vi "test12-LocalExternalStateRegistration.vi"(8 "error in (no error)":errorcluster, 11 "TestCase in":refnum<class "testcase-CSMBroadcast.lvclass">) -> (0 "error out":errorcluster, 3 "TestCase out":refnum<class "testcase-CSMBroadcast.lvclass">)   [LabVIEW 2017, in "testcase-CSMBroadcast.lvclass"]
uses:
  testcase-CSMBroadcast.lvclass
  0b17d103-e67b-41be-a9eb-a2ee1311ff1f.vi
  5999693e-4f8a-4b34-ae87-f34dff5771be.vi
  52a2a10a-a04b-4bad-8df4-e1eb944f47cc.vi
  826f03dd-b4b5-4c6b-9085-8edf6da4f43b.vi
  src/user.lib/_NEVSTOP/Communicable State Machine(CSM)/AdvanceAPI/CSM - Revert Arguments-Safe String.vi
  src/user.lib/_NEVSTOP/Communicable State Machine(CSM)/AdvanceAPI/CSM - Make String Arguments Safe.vi
  src/user.lib/_NEVSTOP/Communicable State Machine(CSM)/AdvanceAPI/CSM - Break Down Multiple States String.vi
  src/user.lib/_NEVSTOP/Communicable State Machine(CSM)/AdvanceAPI/CSM - Keywords.vi
  src/user.lib/_NEVSTOP/Communicable State Machine(CSM)/_Polymophic/CSM - Replace Marks in Messages.vi
  src/user.lib/_NEVSTOP/Communicable State Machine(CSM)/AdvanceAPI/CSM - Get Module Attribute.vi
  src/user.lib/_NEVSTOP/Communicable State Machine(CSM)/_Shared/Trim Single-line Text.vi
  <vilib>/addons/_JKI Toolkits/VI Tester/TestCase.llb/TestCase.lvclass
  src/user.lib/_NEVSTOP/Communicable State Machine(CSM)/Communicable State Machine.lvlib
  CSM/CSM-Testcase.lvlib
  C:/Program Files (x86)/National Instruments/LabVIEW 2017/vi.lib/addons/_JKI Toolkits/VI Tester/TestCase.llb/TestCase.lvclass
panel:
  out "One-Shot Unregistrations":string
  out "One-Shot Registrations":string
  out "LoopCount 2":i32
  out "State History":string
  out "LoopCount":i32
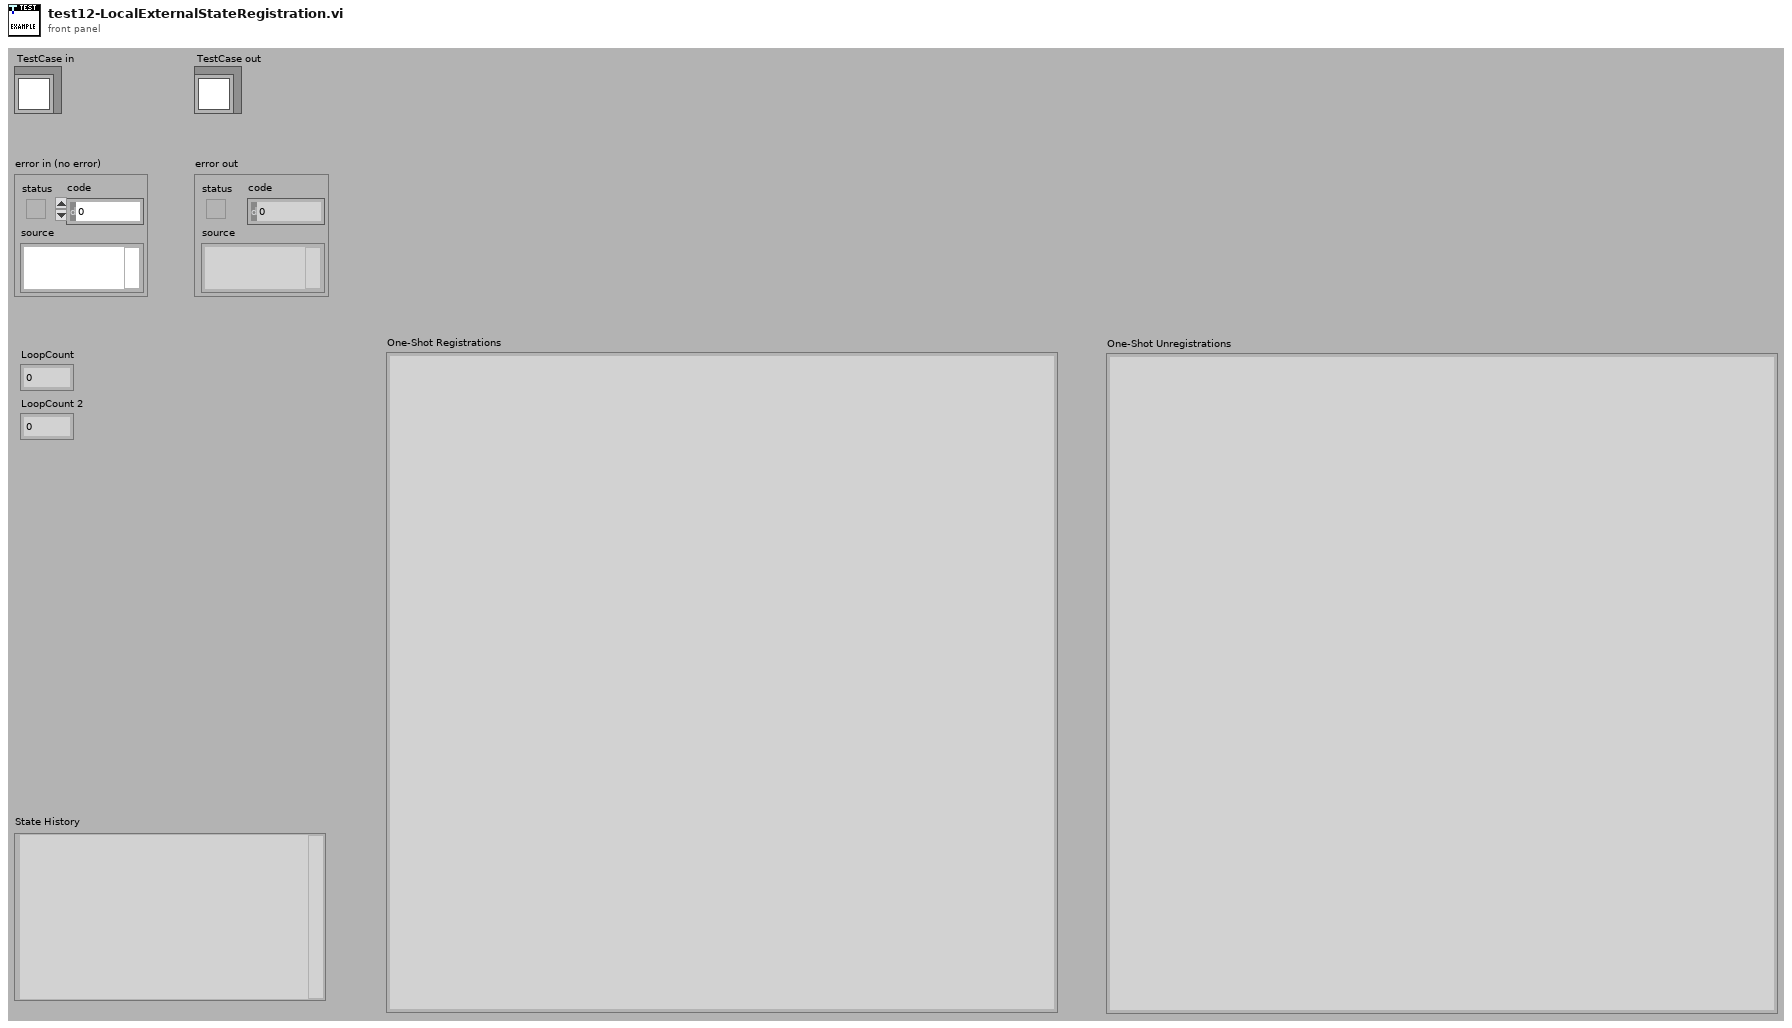
[diagram p1: front panel]
types:
  T1 = enum32{"Invalid", "Standard", "Closed", "Hidden", "Minimized", "Maximized"}
  T2 = enum32{"invalid app kind", "Development System", "Run Time System", "Student Edition", "Embedded LabVIEW", "Evaluation", "Custom"}
  T3 = typedef "Communicable State Machine.lvlib/_CSM_Response Source Message.ctl" = cluster{"‘State":string, "’Arguments":string, "’Error":errorcluster}
  T4 = cluster{"Current VI Reference":refnum<vi>, "Close Panel on Exit?":bool}
  T5 = cluster{"Core":cluster{"Current VI Reference":refnum<vi>, "Close Panel on Exit?":bool}, "Your Boolean data":bool, "Your string data":string}
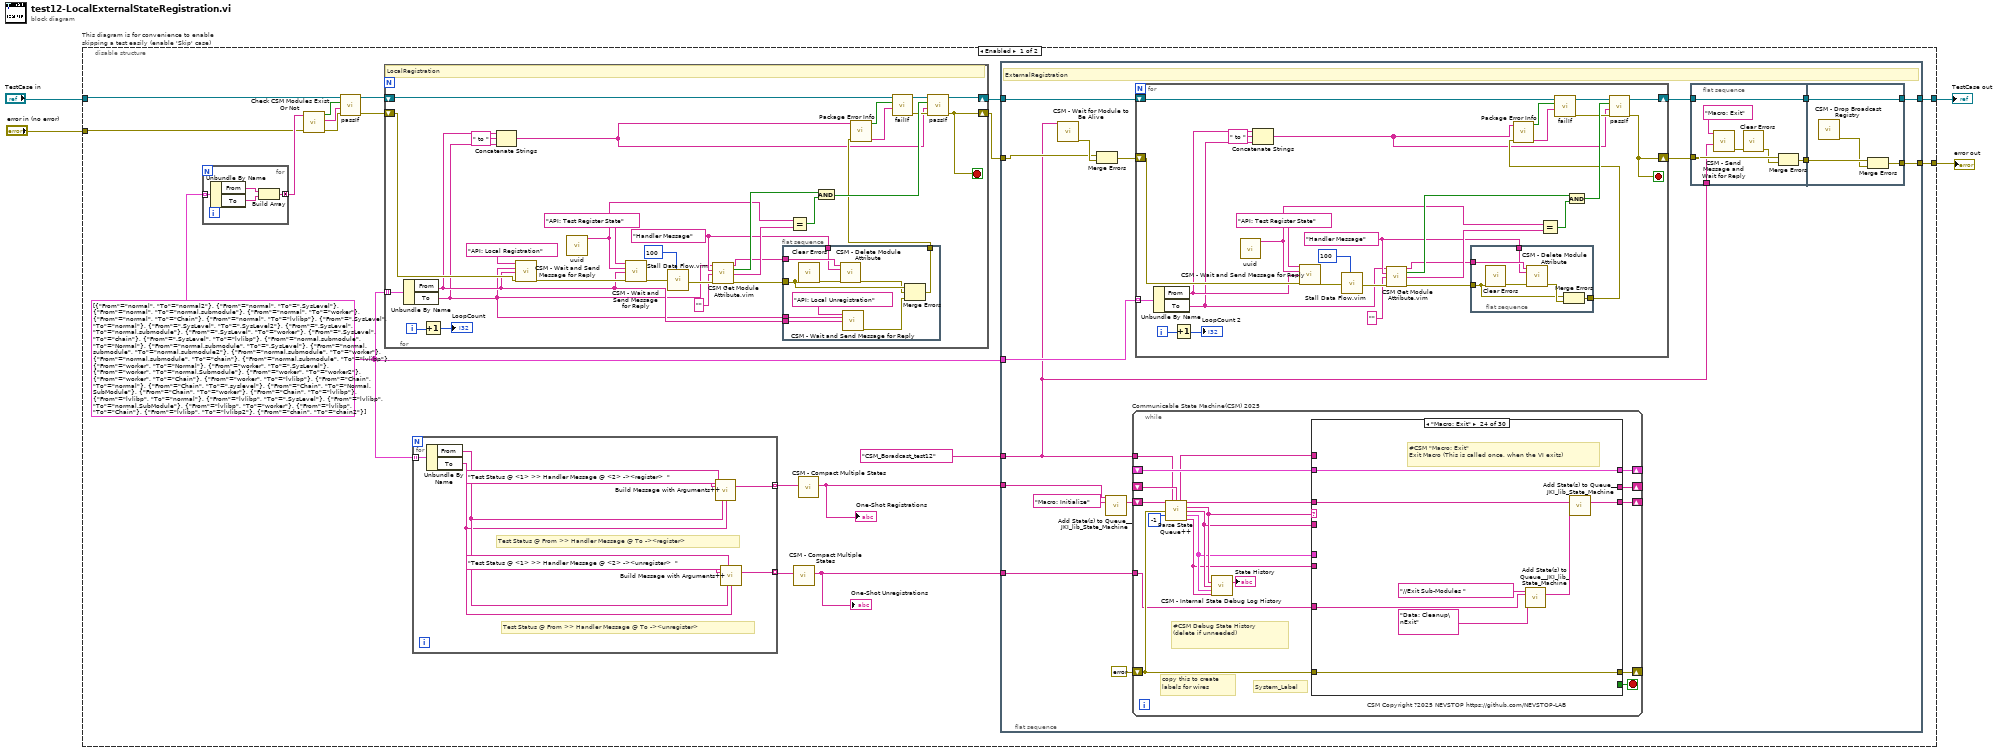
[diagram p0: block diagram]
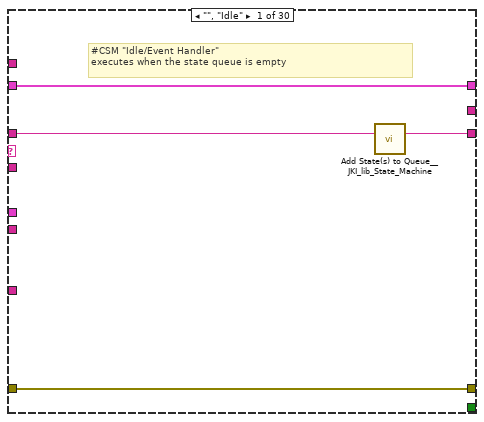
[diagram p2: hidden frame]
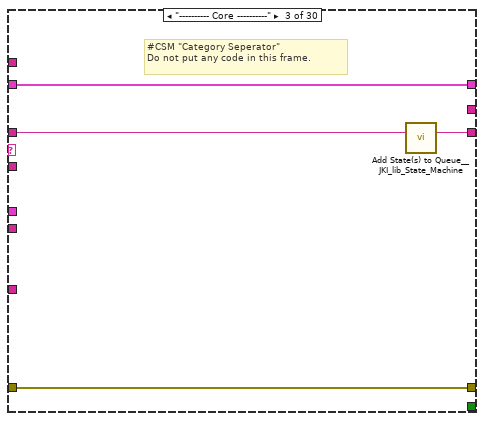
[diagram p4: hidden frame]
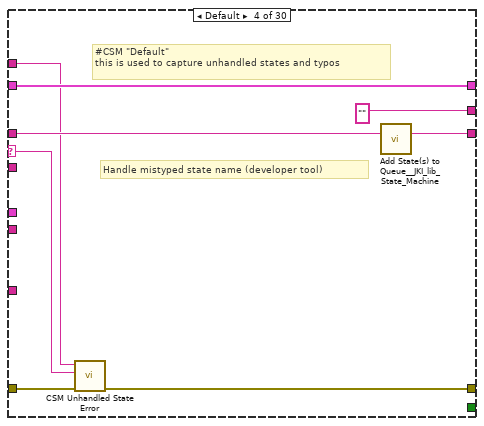
[diagram p5: hidden frame]
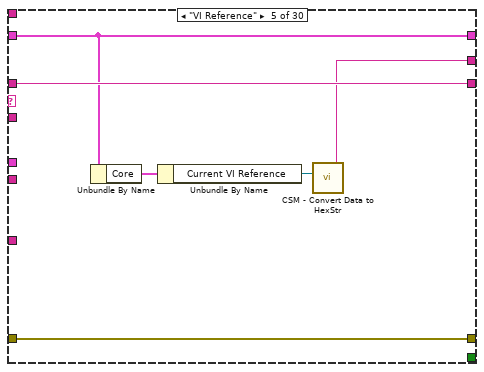
[diagram p6: hidden frame]
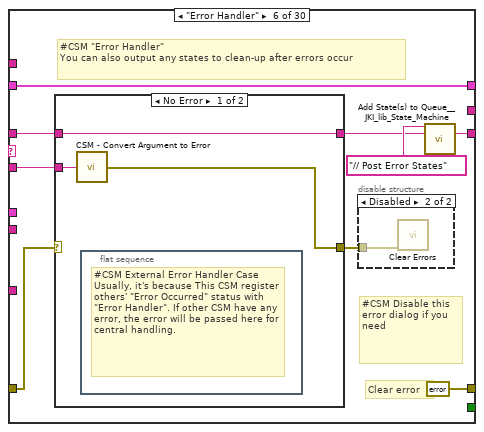
[diagram p7: hidden frame]
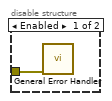
[diagram p8: hidden frame]
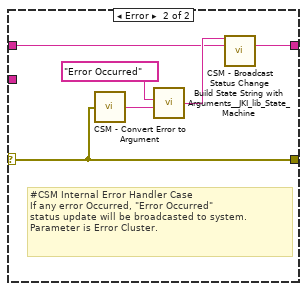
[diagram p9: hidden frame]
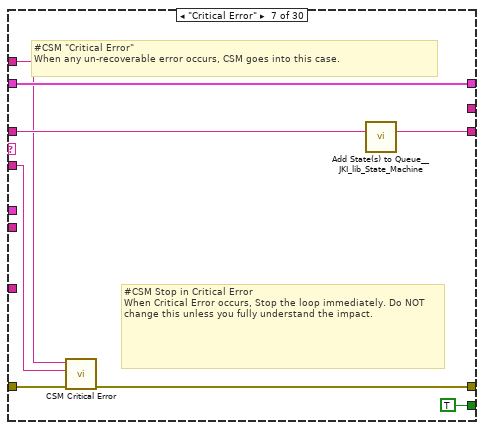
[diagram p10: hidden frame]
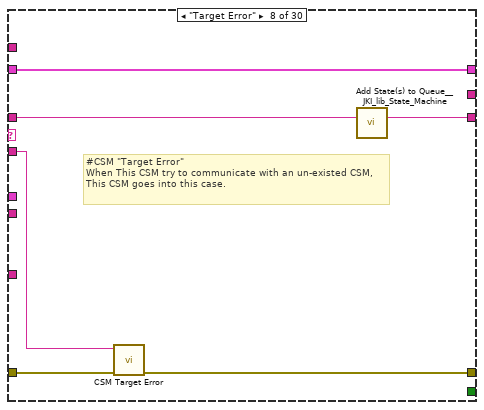
[diagram p11: hidden frame]
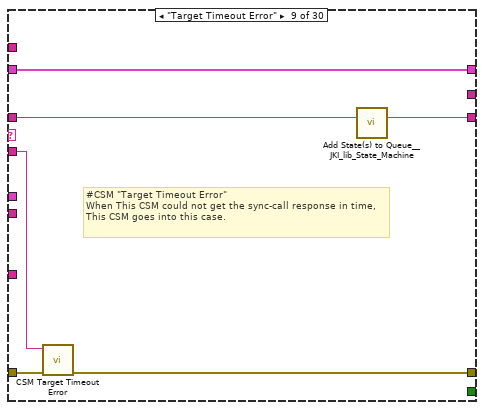
[diagram p12: hidden frame]
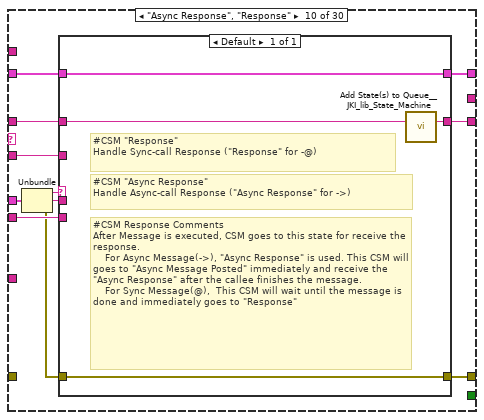
[diagram p13: hidden frame]
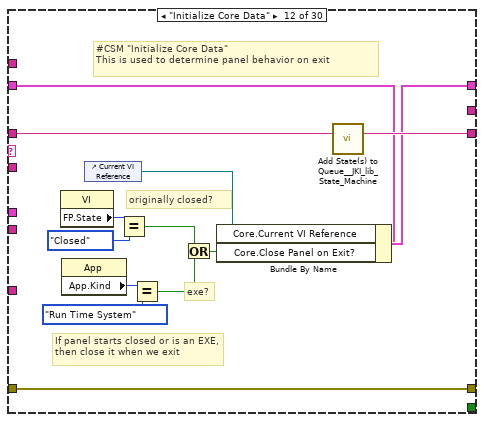
[diagram p15: hidden frame]
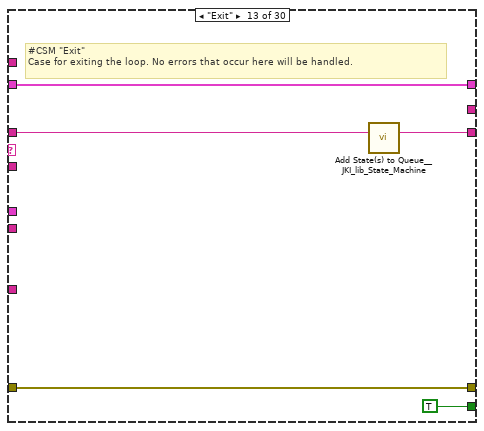
[diagram p16: hidden frame]
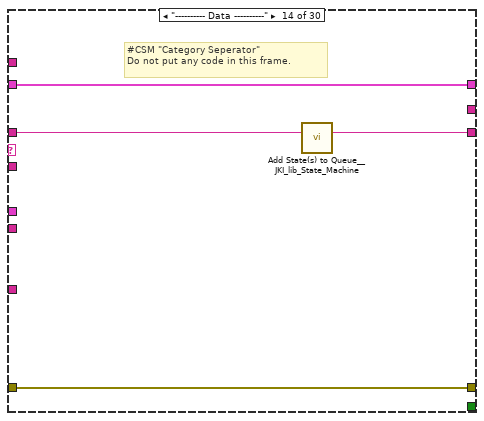
[diagram p17: hidden frame]
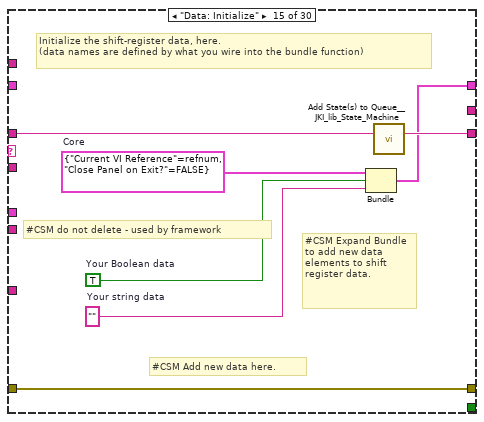
[diagram p18: hidden frame]
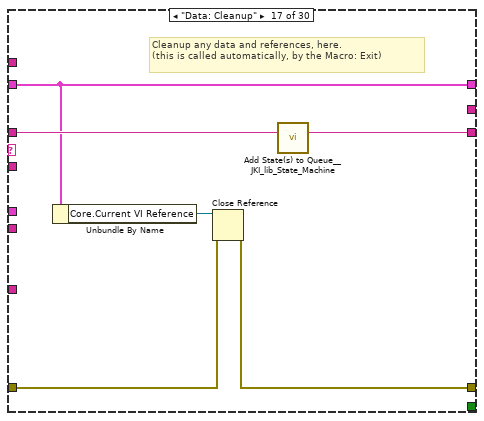
[diagram p20: hidden frame]
diagram:
  n1 = disable-structure "This diagram is for convenience to enable skipping a test easily (enable 'Skip' case)" shown="Enabled" {
    disable-tunnel: "TestCase in" -> [w10 w418]
    disable-tunnel: [w6 w416] -> w1
    disable-tunnel: [w16 w417] -> w3
    disable-tunnel: "error in (no error)" -> [w7 w415]
    frame Enabled {
      w11 = cluster{"From":string, "To":string}[] [{"From"="normal", "To"="normal2"}, {"From"="normal", "To"=".SysLevel"}, {"From"="normal", "To"="normal.submodule"}, {"From"="normal", "To"="worker"}, {"From"="normal", "To"="Chain"}, {"From"="normal", "To"="lvlibp"}, {"From"=".SysLevel", "To"="normal"}, {"From"=".SysLevel", "To"=".SysLevel2"}, {"From"=".SysLevel", "To"="normal.submodule"}, {"From"=".SysLevel", "To"="worker"}, {"From"=".SysLevel", "To"="chain"}, {"From"=".SysLevel", "To"="lvlibp"}, {"From"="normal.submodule", "To"="Normal"}, {"From"="normal.submodule", "To"=".SysLevel"}, {"From"="normal.submodule", "To"="normal.submodule2"}, {"From"="normal.submodule", "To"="worker"}, {"From"="normal.submodule", "To"="chain"}, {"From"="normal.submodule", "To"="lvlibp"}, {"From"="worker", "To"="Normal"}, {"From"="worker", "To"=".SysLevel"}, {"From"="worker", "To"="normal.Submodule"}, {"From"="worker", "To"="worker2"}, {"From"="worker", "To"="Chain"}, {"From"="worker", "To"="lvlibp"}, {"From"="Chain", "To"="normal"}, {"From"="Chain", "To"=".syslevel"}, {"From"="Chain", "To"="Normal.SubModule"}, {"From"="Chain", "To"="worker"}, {"From"="Chain", "To"="lvlibp"}, {"From"="lvlibp", "To"="normal"}, {"From"="lvlibp", "To"=".SysLevel"}, {"From"="lvlibp", "To"="normal.SubModule"}, {"From"="lvlibp", "To"="worker"}, {"From"="lvlibp", "To"="Chain"}, {"From"="lvlibp", "To"="lvlibp2"}, {"From"="chain", "To"="chain2"}]
      n2 = for {
        tunnel: w11 -> [w26] mode=indexing
        tunnel: [w23] -> w14 mode=concatenating
        n3 = Unbundle By Name(w26) -> ("From"=w25:string, "To"=w24:string)
        n4 = Build Array(w25, w24) -> (w23:string[])
      }
      n5 = call "Check CSM Modules Exist Or Not.vi"("error in"=w7, "CSM names in"=w14) -> ("error out"=w12:errorcluster, "Debug string"=w13:string, "All Modules Exist?"=w15:bool)  [unwired: 7 in]
      n6 = call-dynamic "passIf.vi"("error in (no error)"=w12, "message (\"\")"=w13, "pass"=w15, "TestCase in"=w10) -> ("error out"=w8:errorcluster, "TestCase out"=w9:refnum<class "testcase-CSMBroadcast.lvclass">)  [unwired: 6 in]
      n7 = for {
        shift-right: [w37] -> w21
        shift-left: w8 -> [w38]
        shift-right: [w44] -> w22
        shift-left: w9 -> [w34]
        tunnel: w11 -> [w55] mode=indexing
        i -> [w57]
        stop <- w37 stop-if-true
        w39 = "Handler Message" ("To")
        # "LocalRegistration"
        n8 = Unbundle By Name(w55) -> ("From"=w30:string, "To"=w29:string)
        n9 = Increment(x=w57) -> (x+1=→"LoopCount":i32)
        n10 = Concatenate Strings(w30, " to " ("string"), w29) -> (w27:string)
        n11 = call "CSM - Wait and Send Message for Reply.vi"("State"="API: Local Registration", "Arguments (\"\")"=w29, "Target Module"=w30, "Error In (No Error)"=w38) -> ("error out"=w52:errorcluster)  [unwired: 8 in, 3 out]
        n12 = call "uuid.vi"() -> ("UUID"=w46:string)  [unwired: 11 in]
        n13 = call "CSM - Wait and Send Message for Reply.vi"("State"="API: Test Register State", "Arguments (\"\")"=w46, "Target Module"=w30, "Error In (No Error)"=w52) -> ("error out"=w51:errorcluster)  [unwired: 8 in, 3 out]
        n14 = call "Stall Data Flow.vim"("value in"=w51, "milliseconds to wait"=u32 100) -> ("value out"=w49:errorcluster)  [unwired: 1 out]
        n15 = call "CSM Get Module Attribute.vim"("CSM Name"=w29, "Attribute"=w39, "Default Value (Empty Variant)"="", "Error In"=w49) -> ("CSM Name (Dup)"=w40:string, "Found"=w48:bool, "Value"=w45:string, "error out"=w41:errorcluster)  [unwired: 7 in, 1 out]
        n16 = flat-sequence {
          tunnel: w41 -> [w61]
          tunnel: w40 -> [w66]
          tunnel: w39 -> [w65]
          tunnel: w29 -> [w63]
          tunnel: w30 -> [w62]
          tunnel: [w58] -> w31
          frame #0 {
            n17 = call <vilib>:"Clear Errors.vi"("error in (no error)"=w61) -> ("error out"=w67:errorcluster)  [unwired: 5 in, 1 out]
            n18 = call "CSM - Delete Module Attribute.vi"("CSM Name"=w66, "Attribute"=w65, "Error In"=w67) -> ("error out"=w60:errorcluster)  [unwired: 9 in, 3 out]
            n19 = call "CSM - Wait and Send Message for Reply.vi"("State"="API: Local Unregistration", "Arguments (\"\")"=w63, "Target Module"=w62) -> ("error out"=w59:errorcluster)  [unwired: 9 in, 3 out]
            n20 = Merge Errors(w61, w60, w59) -> (w58:errorcluster)
          }
        }
        n21 = Equal?(x=w46, y=w45) -> (x = y?=w43:bool)
        n22 = And(x=w48, y=w43) -> (x .and. y?=w42:bool)
        n23 = call "Package Error Info.vi"("error in"=w31, "String in"=w27) -> ("packed error info out"=w35:string, "error status"=w36:bool)  [unwired: 8 in]
        n24 = call-dynamic "failIf.vi"("message (\"\")"=w35, "fail"=w36, "TestCase in"=w34) -> ("error out"=w32:errorcluster, "TestCase out"=w33:refnum<class "testcase-CSMBroadcast.lvclass">)  [unwired: 7 in]
        n25 = call-dynamic "passIf.vi"("error in (no error)"=w32, "message (\"\")"=w27, "pass"=w42, "TestCase in"=w33) -> ("error out"=w37:errorcluster, "TestCase out"=w44:refnum<class "testcase-CSMBroadcast.lvclass">)  [unwired: 6 in]
      }
      n26 = for {
        tunnel: w11 -> [w73] mode=indexing
        tunnel: [w72] -> w20 mode=indexing
        tunnel: [w68] -> w18 mode=indexing
        # "Test Status @ From >> Handler Message @ To -><unregister>"
        # "Test Status @ From >> Handler Message @ To -><register>"
        n27 = Unbundle By Name(w73) -> ("From"=w70:string, "To"=w69:string)
        n28 = call-poly "Build Message with Arguments++.vi"("States With Replace Token"="Test Status @ <1> >> Handler Message @ <2> -><register>  " ("State"), "<1>"=w70, "<2>"=w69) -> ("States"=w72:string)  [unwired: 12 in]
        n29 = call-poly "Build Message with Arguments++.vi"("States With Replace Token"="Test Status @ <1> >> Handler Message @ <2> -><unregister>  " ("State"), "<1>"=w70, "<2>"=w69) -> ("States"=w68:string)  [unwired: 12 in]
      }
      n30 = call "CSM - Compact Multiple States.vi"("Multiple States"=w18) -> ("States"=w17:string)  [unwired: 9 in]
      "One-Shot Unregistrations" <- w17
      n31 = call "CSM - Compact Multiple States.vi"("Multiple States"=w20) -> ("States"=w19:string)  [unwired: 9 in]
      "One-Shot Registrations" <- w19
      n32 = flat-sequence {
        tunnel: w22 -> [w88]
        tunnel: w21 -> [w82]
        tunnel: w11 -> [w87]
        tunnel: w19 -> [w85]
        tunnel: w17 -> [w81]
        tunnel: [w79] -> w16
        tunnel: [w76] -> w6
        tunnel: "CSM_Boradcast_test12" ("Name (\"\" to Use UUID)") -> [w75]
        frame #0 {
          # "ExternalRegistration"
          n33 = call "CSM - Wait for Module to Be Alive.vi"("CSM Name"=w75) -> ("error out"=w86:errorcluster)  [unwired: 12 in, 2 out]
          n34 = Merge Errors(w82, w86) -> (w83:errorcluster)
          n35 = call <vilib>:"Add State(s) to Queue__JKI_lib_State_Machine.vi"("State(s) in Front (\"\")"=w85, "State(s) in (\"\")"="Macro: Initialize" ("Init State(\"Macro: Initialize\")")) -> ("States Out"=w89:string)  [unwired: 13 in]
          n36 = while "Communicable State Machine(CSM) 2025" {
            shift-right: [w151] -> _
            shift-left: _ -> [w150]
            shift-right: [w154] -> _
            shift-left: errorcluster {"status"=FALSE, "code"=0, "source"=""} ("error out") -> [w149]
            shift-right: [w153] -> _
            shift-left: w89 -> [w155]
            shift-right: [w148] -> _
            shift-left: _ -> [w142]
            tunnel: w81 -> [w139]
            tunnel: w75 -> [w138]
            stop <- w152 stop-if-true
            # "#CSM Debug State History\n(delete if unneeded)"
            # "copy this to create labels for wires"
            # "System_Label"
            # "CSM Copyright ?2025 NEVSTOP https://github.com/NEVSTOP-LAB"
            n37 = call "Parse State Queue++.vi"("State Queue"=w155, "Name (\"\" to Use UUID)"=w138, "Response Arguments"=w142, "Previous Error"=w149, "Dequeue (1 ms)"=-1 ("Timeout")) -> ("Name Used"=w143:string, "Remaining States"=w156:string, "Current State"=w147:string, "Arguments"=w146:string, "Additional Information"=w145:T3, "Source CSM"=w144:string)  [unwired: 5 in]
            n38 = call "CSM - Internal State Debug Log History.vi"("State"=w147, "Arguments (\"\")"=w146, ">> Response Source Message >>"=w145, "Source (\"\")"=w144) -> ("Debug Log"=→"State History":string)  [unwired: 11 in]
            n39 = case shown="\"Macro: Exit\"" w147 {
              selector: w147 -> [_ _ _ w170 _ _ _ _ _ _ _ _ _ _ _ _ _ _ _ _ _ _ _ _ _ _ _ _ _ _]
              tunnel: w156 -> [w157 w162 w167 w174 w180 w186 w207 w213 w219 w227 w238 w252 w257 w261 w268 w270 w277 w281 w285 w291 w306 w375 w380 w388 w390 w394 w399 w406 w410 w414]
              tunnel: w146 -> [_ _ _ _ _ w185 w203 w212 w217 w226 _ _ _ _ _ _ _ _ _ w286 w300 _ _ _ _ _ w397 _ _ _]
              tunnel: w150 -> [w158 w161 w164 w172 w179 w189 w208 w214 w220 w229 w237 w245 w255 w258 _ w269 w272 w278 w283 w289 w302 w372 w377 w385 w389 w393 w398 w403 w407 w411]
              tunnel: [w159 w163 w165 w168 w181 errorcluster {"status"=FALSE, "code"=0, "source"=""} ("error out") w204 w210 w216 w232 w239 w249 w254 w259 w265 w271 w273 w279 w282 w287 w303 w373 w378 w386 w391 w395 w400 w404 w408 w412] -> w154
              tunnel: w149 -> [w159 w163 w165 w175 w181 w187 w209 w211 w218 _ w239 w249 w254 w259 w265 w271 w274 w279 w282 w288 w304 w373 w378 w386 w391 w395 w400 w404 w408 w412]
              tunnel: [w160 w162 w166 w173 w180 w182 w206 w215 w221 w228 w238 w251 w256 w260 w267 w270 w276 w280 w284 w290 w305 w374 w379 w387 w390 w394 w399 w405 w409 w413] -> w153
              tunnel: [_ _ _ _ _ _ TRUE _ _ _ _ _ TRUE _ _ _ _ _ _ _ _ _ _ _ _ _ _ _ _ _] -> w152
              tunnel: [w158 w161 w164 w172 w179 w189 w208 w214 w220 w230 w237 w250 w255 w258 w266 w269 w272 w278 w283 w289 w302 w372 w377 w385 w389 w393 w398 w403 w407 w411] -> w151
              tunnel: w144 -> [_ _ _ _ _ _ _ _ _ w224 _ _ _ _ _ _ _ _ _ _ _ _ _ _ _ _ _ _ _ _]
              tunnel: w145 -> [_ _ _ _ _ _ _ _ _ w231 _ _ _ _ _ _ _ _ _ _ _ _ _ _ _ _ _ _ _ _]
              tunnel: [_ _ _ "" w176 _ _ _ _ _ _ _ _ _ _ _ _ _ _ _ _ _ _ _ _ "API1 Response" w396 _ _ _] -> w148
              tunnel: w143 -> [_ _ _ w169 _ _ w202 _ _ _ _ _ _ _ _ _ _ _ _ _ _ _ _ _ _ _ _ _ _ _]
              tunnel: w139 -> [_ _ _ _ _ _ _ _ _ _ _ _ _ _ _ _ _ _ _ _ _ _ _ w381 _ _ _ _ _ _]
              frame "", "Idle" {
                # "#CSM \"Idle/Event Handler\"\nexecutes when the state queue is empty"
                n40 = call <vilib>:"Add State(s) to Queue__JKI_lib_State_Machine.vi"("State(s) in (\"\")"=w157) -> ("States Out"=w160:string)  [unwired: 14 in]
              }
              frame "CSM Documentation" {
                # "#CSM README FIRST\n\nCommunicable State Machine(CSM) is a LabVIEW application framework that builds upon JKI State Machine(JKISM). It follows the pattern of JKISM and extends the keywords to describe message communication between modules, including concepts such as Sync-Message, Async-Message, Subscription/Unsubscription of status - essential elements for creating reusable code modules. For more information, please visit the CSM wiki: https://nevstop-lab.github.io/CSM-Wiki/\n\nFor instructions on JKI State Machine, visit: http://jki.net/state-machine/\nFor information about CSM, visit: https://github.com/NEVSTOP-LAB"
                # "#CSM \"Documentation\"\nCase for holding CSM Documenation"
              }
              frame "---------- Core ----------" {
                # "#CSM \"Category Seperator\"\nDo not put any code in this frame."
                n41 = call <vilib>:"Add State(s) to Queue__JKI_lib_State_Machine.vi"("State(s) in (\"\")"=w167) -> ("States Out"=w166:string)  [unwired: 14 in]
              }
              frame Default {
                # "#CSM \"Default\"\nthis is used to capture unhandled states and typos"
                # "Handle mistyped state name (developer tool)"
                n42 = call "CSM Unhandled State Error.vi"("error in (no error)"=w175, "Undefined State"=w170, "CSM Name"=w169) -> ("error out"=w168:errorcluster)  [unwired: 8 in]
                n43 = call <vilib>:"Add State(s) to Queue__JKI_lib_State_Machine.vi"("State(s) in (\"\")"=w174) -> ("States Out"=w173:string)  [unwired: 14 in]
              }
              frame "VI Reference" {
                n44 = Unbundle By Name(w179) -> ("Core"=w178:T4)
                n45 = Unbundle By Name(w178) -> ("Current VI Reference"=w177:refnum<vi>)
                n46 = call "CSM - Convert Data to HexStr.vi"("Variant"=w177) -> ("HEX String (0-9,A-F)"=w176:string)  [unwired: 8 in]
              }
              frame "Error Handler" {
                # "#CSM Disable this error dialog if you need"
                # "#CSM \"Error Handler\"\nYou can also output any states to clean-up after errors occur"
                # "Clear error"
                n47 = case shown="No Error" w187 {
                  selector: w187 -> [_ w196]
                  tunnel: [w195 w198] -> w183
                  tunnel: w186 -> [w195 w197]
                  tunnel: w185 -> [w194 _]
                  tunnel: [w193 w196] -> w188
                  frame No Error {
                    n48 = call "CSM - Convert Argument to Error.vi"("Argument"=w194) -> ("Error"=w193:errorcluster)  [unwired: 4 in]
                    n49 = flat-sequence {
                      frame #0 {
                        # "#CSM External Error Handler Case\nUsually, it's because This CSM register others' \"Error Occurred\" status with \"Error Handler\". If other CSM have any error, the error will be passed here for central handling."
                      }
                    }
                  }
                  frame Error {
                    # "#CSM Internal Error Handler Case \nIf any error Occurred, \"Error Occurred\" \nstatus update will be broadcasted to system.\nParameter is Error Cluster."
                    n50 = call "CSM - Convert Error to Argument.vi"("Error"=w196) -> ("Argument"=w200:string)  [unwired: 4 in]
                    n51 = call <vilib>:"Build State String with Arguments__JKI_lib_State_Machine.vi"("Arguments (\"\")"=w200, "State"="Error Occurred" ("Status with Arguments")) -> ("State with Arguments"=w199:string)  [unwired: 4 in]
                    n52 = call "CSM - Broadcast Status Change.vi"("Status With Arguments"=w199, "State Queue"=w197) -> ("Remaining States"=w198:string)  [unwired: 13 in]
                  }
                }
                n53 = disable-structure shown="Disabled" {
                  disable-tunnel: w188 -> [w191 w192]
                  frame Enabled {
                    n54 = call <vilib>:"General Error Handler.vi"("error in (no error)"=w191) -> ()  [unwired: 10 in, 5 out]
                  }
                  frame Disabled {
                    n55 = call <vilib>:"Clear Errors.vi"("error in (no error)"=w192) -> ()  [unwired: 5 in, 2 out]
                  }
                }
                n56 = call <vilib>:"Add State(s) to Queue__JKI_lib_State_Machine.vi"("State(s) in Front (\"\")"="// Post Error States", "State(s) in (\"\")"=w183) -> ("States Out"=w182:string)  [unwired: 13 in]
              }
              frame "Critical Error" {
                # "#CSM Stop in Critical Error\nWhen Critical Error occurs, Stop the loop immediately. Do NOT change this unless you fully understand the impact."
                # "#CSM \"Critical Error\"\nWhen any un-recoverable error occurs, CSM goes into this case."
                n57 = call "CSM Critical Error.vi"("error in (no error)"=w209, "Arugments (As Reason)"=w203, "CSM Name"=w202) -> ("error out"=w204:errorcluster)  [unwired: 8 in]
                n58 = call <vilib>:"Add State(s) to Queue__JKI_lib_State_Machine.vi"("State(s) in (\"\")"=w207) -> ("States Out"=w206:string)  [unwired: 14 in]
              }
              frame "Target Error" {
                # "#CSM \"Target Error\"\nWhen This CSM try to communicate with an un-existed CSM, This CSM goes into this case."
                n59 = call "CSM Target Error.vi"("error in (no error)"=w211, "Arguments (As CSM Name)"=w212) -> ("error out"=w210:errorcluster)  [unwired: 9 in]
                n60 = call <vilib>:"Add State(s) to Queue__JKI_lib_State_Machine.vi"("State(s) in (\"\")"=w213) -> ("States Out"=w215:string)  [unwired: 14 in]
              }
              frame "Target Timeout Error" {
                # "#CSM \"Target Timeout Error\"\nWhen This CSM could not get the sync-call response in time, This CSM goes into this case."
                n61 = call "CSM Target Timeout Error.vi"("error in (no error)"=w218, "Arguments (As CSM Name)"=w217) -> ("error out"=w216:errorcluster)  [unwired: 9 in]
                n62 = call <vilib>:"Add State(s) to Queue__JKI_lib_State_Machine.vi"("State(s) in (\"\")"=w219) -> ("States Out"=w221:string)  [unwired: 14 in]
              }
              frame "Async Response", "Response" {
                n63 = Unbundle(w231) -> ("‘State"=w225:string, "’Arguments"=w223:string, "’Error"=w222:errorcluster)
                n64 = case shown="Default" w225 {
                  tunnel: [w236] -> w232
                  tunnel: w222 -> [w236]
                  tunnel: [w235] -> w230
                  tunnel: w229 -> [w235]
                  tunnel: [w233] -> w228
                  tunnel: w227 -> [w234]
                  tunnel: w226 -> [_]
                  tunnel: w224 -> [_]
                  tunnel: w223 -> [_]
                  frame Default {
                    # "#CSM Response Comments\nAfter Message is executed, CSM goes to this state for receive the response.\n    For Async Message(->), \"Async Response\" is used. This CSM will goes to \"Async Message Posted\" immediately and receive the \"Async Response\" after the callee finishes the message.\n    For Sync Message(@),  This CSM will wait until the message is done and immediately goes to \"Response\""
                    # "#CSM \"Async Response\"\nHandle Async-call Response (\"Async Response\" for ->)"
                    # "#CSM \"Response\"\nHandle Sync-call Response (\"Response\" for -@)"
                    n65 = call <vilib>:"Add State(s) to Queue__JKI_lib_State_Machine.vi"("State(s) in (\"\")"=w234) -> ("States Out"=w233:string)  [unwired: 14 in]
                  }
                }
              }
              frame "Async Message Posted" {
                # "#CSM \"Async Message Posted\"\nAfter Async Message is posted (-> or ->| ), CSM goes to this state for post-action.\nYou can use Argument - State to tell which Async Message is called."
              }
              frame "Initialize Core Data" {
                # "#CSM \"Initialize Core Data\"\nThis is used to determine panel behavior on exit"
                # "originally closed?"
                # "exe?"
                # "If panel starts closed or is an EXE, then close it when we exit"
                n66 = property class="VI"() -> ("FP.State"=w242:T1)  [unwired: 2 in, 2 out]
                n67 = property class="App"() -> ("App.Kind"=w248:T2)  [unwired: 2 in, 2 out]
                n68 = control-ref of="Current VI Reference"() -> (w243:refnum<vi>)
                n69 = Equal?(x=w242, y=T1."Closed" ("Front Panel Window:State")) -> (x = y?=w240:bool)
                n70 = Equal?(x=w248, y=T2."Run Time System" ("Application:Kind")) -> (x = y?=w246:bool)
                n71 = Or(x=w240, y=w246) -> (x .or. y?=w244:bool)
                n72 = Bundle By Name(cluster=w245, "Core.Current VI Reference"=w243, "Core.Close Panel on Exit?"=w244) -> (w250:T5)
                n73 = call <vilib>:"Add State(s) to Queue__JKI_lib_State_Machine.vi"("State(s) in (\"\")"=w252) -> ("States Out"=w251:string)  [unwired: 14 in]
              }
              frame "Exit" {
                # "#CSM \"Exit\"\nCase for exiting the loop. No errors that occur here will be handled."
                n74 = call <vilib>:"Add State(s) to Queue__JKI_lib_State_Machine.vi"("State(s) in (\"\")"=w257) -> ("States Out"=w256:string)  [unwired: 14 in]
              }
              frame "---------- Data ----------" {
                # "#CSM \"Category Seperator\"\nDo not put any code in this frame."
                n75 = call <vilib>:"Add State(s) to Queue__JKI_lib_State_Machine.vi"("State(s) in (\"\")"=w261) -> ("States Out"=w260:string)  [unwired: 14 in]
              }
              frame "Data: Initialize" {
                w262 = T4 {"Current VI Reference"=refnum, "Close Panel on Exit?"=FALSE}  # Core
                w264 = TRUE  # Your Boolean data
                w263 = ""  # Your string data
                # "#CSM do not delete - used by framework"
                # "#CSM Expand Bundle to add new data elements to shift register data."
                # "#CSM Add new data here."
                # "Initialize the shift-register data, here.\n(data names are defined by what you wire into the bundle function)"
                n76 = Bundle("Core"=w262, "Your Boolean data"=w264, "Your string data"=w263) -> (w266:T5)  [unwired: 1 in]
                n77 = call <vilib>:"Add State(s) to Queue__JKI_lib_State_Machine.vi"("State(s) in (\"\")"=w268) -> ("States Out"=w267:string)  [unwired: 14 in]
              }
              frame "Data: Update Indicators" {
              }
              frame "Data: Cleanup" {
                # "Cleanup any data and references, here.\n(this is called automatically, by the Macro: Exit)"
                n78 = Unbundle By Name(w272) -> ("Core.Current VI Reference"=w275:refnum<vi>)
                n79 = Close Reference(reference=w275, error in (no error)=w274) -> (error out=w273:errorcluster)
                n80 = call <vilib>:"Add State(s) to Queue__JKI_lib_State_Machine.vi"("State(s) in (\"\")"=w277) -> ("States Out"=w276:string)  [unwired: 14 in]
              }
              frame "---------- UI ----------" {
                # "#CSM \"Category Seperator\"\nDo not put any code in this frame."
                n81 = call <vilib>:"Add State(s) to Queue__JKI_lib_State_Machine.vi"("State(s) in (\"\")"=w281) -> ("States Out"=w280:string)  [unwired: 14 in]
              }
              frame "UI: Initialize" {
                # "#CSM \"UI: Initialize\"\nInitialize the User Interface, here.\n(this is called automatically, by the Macro: Init)"
                n82 = call <vilib>:"Add State(s) to Queue__JKI_lib_State_Machine.vi"("State(s) in (\"\")"=w285) -> ("States Out"=w284:string)  [unwired: 14 in]
              }
              frame "UI: Cursor Set" {
                # "#CSM \"UI: Cursor Set\"\nSet and Unset Cursor Busy.\n(Usage: \"UI: Cursor Set >> Busy|Idle\")"
                # "Argument"
                n83 = disable-structure shown="TARGET_TYPE!=Windows" {
                  disable-tunnel: w288 -> [w294 w299]
                  disable-tunnel: [w293 w299] -> w287
                  disable-tunnel: w286 -> [w292 _]
                  frame condition #0 (active) {
                    n84 = case shown="\"Idle\", Default" w292 {
                      tunnel: w294 -> [w296 w298]
                      tunnel: [w295 w297] -> w293
                      frame "Idle", Default {
                        n85 = call <vilib>:"Unset Busy.vi"("error in (no error)"=w296) -> ("error out"=w295:errorcluster)  [unwired: 10 in]
                      }
                      frame "Busy" {
                        n86 = call <vilib>:"Set Busy.vi"("error in (no error)"=w298) -> ("error out"=w297:errorcluster)  [unwired: 9 in, 1 out]
                      }
                    }
                  }
                  frame condition #1 {
                  }
                }
                n87 = call <vilib>:"Add State(s) to Queue__JKI_lib_State_Machine.vi"("State(s) in (\"\")"=w291) -> ("States Out"=w290:string)  [unwired: 14 in]
              }
              frame "UI: Front Panel State" {
                # "#CSM \"UI: Front Panel State\"\nSet Front Panel Open or Closed\n(Usage: \"UI: Front Panel State >> Open|Close\")"
                # "Argument"
                n88 = Unbundle By Name(w302) -> ("Core.Current VI Reference"=w301:refnum<vi>)
                n89 = call <vilib>:"Add State(s) to Queue__JKI_lib_State_Machine.vi"("State(s) in (\"\")"=w306) -> ("States Out"=w305:string)  [unwired: 14 in]
                n90 = case shown="\"Close\", \"Closed\"" w300 {
                  tunnel: w304 -> [w312 w327 w338 w351 w364]
                  tunnel: [w314 w328 w340 w353 w366] -> w303
                  tunnel: w301 -> [w313 w325 w339 w352 w365]
                  frame "Open", "Standard", Default {
                    w307 = T1."Standard" ("State")
                    n91 = property class="VI"(reference=w313, error in=w312) -> (reference out=w310:refnum<vi>, error out=w311:errorcluster, "FP.State"=w309:T1)
                    n92 = Not Equal?(x=w309, y=w307) -> (x != y?=w308:bool)
                    n93 = case shown="True" w308 {
                      tunnel: [w318 w320] -> w314
                      tunnel: w311 -> [w317 w320]
                      tunnel: w310 -> [w316 _]
                      tunnel: w307 -> [w315 _]
                      frame True {
                        n94 = invoke class="VI" method="FP.Open"(reference=w316, error in=w317, "Activate"=TRUE, "State"=w315) -> (error out=w318:errorcluster)  [unwired: 1 in, 4 out]
                      }
                      frame False {
                      }
                    }
                  }
                  frame "Close", "Closed" {
                    n95 = property class="VI"(reference=w325, error in=w327) -> (reference out=w324:refnum<vi>, error out=w326:errorcluster, "FP.State"=w322:T1)
                    n96 = Not Equal?(x=w322, y=T1."Closed" ("Front Panel Window:State")) -> (x != y?=w321:bool)
                    n97 = case shown="False" w321 {
                      tunnel: [w329 w332] -> w328
                      tunnel: w326 -> [w329 w331]
                      tunnel: w324 -> [_ w330]
                      frame False {
                      }
                      frame True {
                        n98 = invoke class="VI" method="FP.Close"(reference=w330, error in=w331) -> (error out=w332:errorcluster)  [unwired: 1 in, 2 out]
                      }
                    }
                  }
                  frame "Hidden", "Hide" {
                    w333 = T1."Hidden" ("State")
                    n99 = property class="VI"(reference=w339, error in=w338) -> (reference out=w336:refnum<vi>, error out=w337:errorcluster, "FP.State"=w335:T1)
                    n100 = Not Equal?(x=w335, y=w333) -> (x != y?=w334:bool)
                    n101 = case shown="True" w334 {
                      tunnel: [w344 w345] -> w340
                      tunnel: w337 -> [w343 w345]
                      tunnel: w336 -> [w342 _]
                      tunnel: w333 -> [w341 _]
                      frame True {
                        n102 = invoke class="VI" method="FP.Open"(reference=w342, error in=w343, "State"=w341) -> (error out=w344:errorcluster)  [unwired: 2 in, 4 out]
                      }
                      frame False {
                      }
                    }
                  }
                  frame "Minimize", "Minimized" {
                    w346 = T1."Minimized" ("State")
                    n103 = property class="VI"(reference=w352, error in=w351) -> (reference out=w349:refnum<vi>, error out=w350:errorcluster, "FP.State"=w348:T1)
                    n104 = Not Equal?(x=w348, y=w346) -> (x != y?=w347:bool)
                    n105 = case shown="True" w347 {
                      tunnel: [w357 w358] -> w353
                      tunnel: w350 -> [w356 w358]
                      tunnel: w349 -> [w355 _]
                      tunnel: w346 -> [w354 _]
                      frame True {
                        n106 = invoke class="VI" method="FP.Open"(reference=w355, error in=w356, "State"=w354) -> (error out=w357:errorcluster)  [unwired: 2 in, 4 out]
                      }
                      frame False {
                      }
                    }
                  }
                  frame "Maximize", "Maximized" {
                    w359 = T1."Maximized" ("State")
                    n107 = property class="VI"(reference=w365, error in=w364) -> (reference out=w362:refnum<vi>, error out=w363:errorcluster, "FP.State"=w361:T1)
                    n108 = Not Equal?(x=w361, y=w359) -> (x != y?=w360:bool)
                    n109 = case shown="True" w360 {
                      tunnel: [w370 w371] -> w366
                      tunnel: w363 -> [w369 w371]
                      tunnel: w362 -> [w368 _]
                      tunnel: w359 -> [w367 _]
                      frame True {
                        n110 = invoke class="VI" method="FP.Open"(reference=w368, error in=w369, "State"=w367) -> (error out=w370:errorcluster)  [unwired: 2 in, 4 out]
                      }
                      frame False {
                      }
                    }
                  }
                }
              }
              frame "---------- Macro ----------" {
                # "#CSM \"Category Seperator\"\nDo not put any code in this frame."
                n111 = call <vilib>:"Add State(s) to Queue__JKI_lib_State_Machine.vi"("State(s) in (\"\")"=w375) -> ("States Out"=w374:string)  [unwired: 14 in]
              }
              frame "Macro: Initialize" {
                # "#CSM \"Macro: Initialize\"\nInitialization Macro (This is called once, when the VI starts)"
                n112 = call <vilib>:"Add State(s) to Queue__JKI_lib_State_Machine.vi"("State(s) in Front (\"\")"="Data: Initialize\nInitialize Core Data\nData: Update Indicators", "State(s) in (\"\")"=w380) -> ("States Out"=w379:string)  [unwired: 13 in]
              }
              frame "Macro: Exit" {
                # "#CSM \"Macro: Exit\"\nExit Macro (This is called once, when the VI exits)"
                n113 = call <vilib>:"Add State(s) to Queue__JKI_lib_State_Machine.vi"("State(s) in Front (\"\")"="//Exit Sub-Modules ", "State(s) in (\"\")"=w381, "State(s) at Back (\"\")"="Data: Cleanup\nExit") -> ("States Out"=w383:string)  [unwired: 12 in]
                n114 = call <vilib>:"Add State(s) to Queue__JKI_lib_State_Machine.vi"("State(s) in Front (\"\")"=w383, "State(s) in (\"\")"=w388) -> ("States Out"=w387:string)  [unwired: 13 in]
              }
              frame "---------- API ----------" {
                # "#CSM \"Category Seperator\"\nDo not put any code in this frame."
              }
              frame "API: API1" {
                # "#CSM API Example\nCopy/Rename this case for your own API"
                # "#CSM Response\nConnect this to return the response of your API"
                # "#CSM >> Msg/Rep's CSM >>\nIf you need to tell who triggered this state , use this string. If it's this case itself, this string is \"\"."
                # "#CSM >> Arguments >>\nDeal with the parameter if any"
              }
              frame "API: API2" {
                # "#CSM API Example\nCopy/Rename this case for your own API"
                # "unpack Hex String  to Variant\nif complex parameter is needed."
                n115 = call "CSM - Convert HexStr to Data.vi"("HEX String"=w397) -> ()  [unwired: 7 in, 2 out]
                n116 = disable-structure shown="Disabled" {
                  disable-tunnel: [w401 "API2 Response"] -> w396
                  frame Disabled {
                    # "pack variant to hexstr \nif complex response is needed."
                    # "complex Response"
                    n117 = call "CSM - Convert Data to HexStr.vi"() -> ("HEX String (0-9,A-F)"=w401:string)  [unwired: 9 in]
                  }
                  frame Enabled {
                  }
                }
              }
              frame "---------- Action ----------" {
                # "#CSM \"Category Seperator\"\nDo not put any code in this frame."
                n118 = call <vilib>:"Add State(s) to Queue__JKI_lib_State_Machine.vi"("State(s) in (\"\")"=w406) -> ("States Out"=w405:string)  [unwired: 14 in]
              }
              frame "Action: action1" {
                # "#CSM \"Internal State\"\nThis category is used for holding internal states"
                n119 = call <vilib>:"Add State(s) to Queue__JKI_lib_State_Machine.vi"("State(s) in (\"\")"=w410) -> ("States Out"=w409:string)  [unwired: 14 in]
              }
              frame "Action: action2" {
                # "#CSM \"Internal State\"\nThis category is used for holding internal states"
                n120 = call <vilib>:"Add State(s) to Queue__JKI_lib_State_Machine.vi"("State(s) in (\"\")"=w414) -> ("States Out"=w413:string)  [unwired: 14 in]
              }
            }
          }
          n121 = for {
            shift-right: [w114] -> w84
            shift-left: w83 -> [w108]
            shift-right: [w120] -> w78
            shift-left: w88 -> [w109]
            tunnel: w87 -> [w129] mode=indexing
            i -> [w131]
            stop <- w114 stop-if-true
            w115 = "Handler Message" ("To")
            n122 = Unbundle By Name(w129) -> ("From"=w105:string, "To"=w104:string)
            n123 = Increment(x=w131) -> (x+1=→"LoopCount 2":i32)
            n124 = call "uuid.vi"() -> ("UUID"=w122:string)  [unwired: 11 in]
            n125 = Concatenate Strings(w105, " to " ("string"), w104) -> (w103:string)
            n126 = call "CSM - Wait and Send Message for Reply.vi"("State"="API: Test Register State", "Arguments (\"\")"=w122, "Target Module"=w105, "Error In (No Error)"=w108) -> ("error out"=w127:errorcluster)  [unwired: 8 in, 3 out]
            n127 = call "Stall Data Flow.vim"("value in"=w127, "milliseconds to wait"=u32 100) -> ("value out"=w125:errorcluster)  [unwired: 1 out]
            n128 = call "CSM Get Module Attribute.vim"("CSM Name"=w104, "Attribute"=w115, "Default Value (Empty Variant)"="", "Error In"=w125) -> ("CSM Name (Dup)"=w116:string, "Found"=w124:bool, "Value"=w121:string, "error out"=w117:errorcluster)  [unwired: 7 in, 1 out]
            n129 = flat-sequence {
              tunnel: w117 -> [w133]
              tunnel: w116 -> [w136]
              tunnel: w115 -> [w135]
              tunnel: [w132] -> w107
              frame #0 {
                n130 = call <vilib>:"Clear Errors.vi"("error in (no error)"=w133) -> ("error out"=w137:errorcluster)  [unwired: 5 in, 1 out]
                n131 = call "CSM - Delete Module Attribute.vi"("CSM Name"=w136, "Attribute"=w135, "Error In"=w137) -> ("error out"=w134:errorcluster)  [unwired: 9 in, 3 out]
                n132 = Merge Errors(w133, w134) -> (w132:errorcluster)
              }
            }
            n133 = call "Package Error Info.vi"("error in"=w107, "String in"=w103) -> ("packed error info out"=w112:string, "error status"=w113:bool)  [unwired: 8 in]
            n134 = Equal?(x=w122, y=w121) -> (x = y?=w119:bool)
            n135 = call-dynamic "failIf.vi"("message (\"\")"=w112, "fail"=w113, "TestCase in"=w109) -> ("error out"=w110:errorcluster, "TestCase out"=w111:refnum<class "testcase-CSMBroadcast.lvclass">)  [unwired: 7 in]
            n136 = And(x=w124, y=w119) -> (x .and. y?=w118:bool)
            n137 = call-dynamic "passIf.vi"("error in (no error)"=w110, "message (\"\")"=w103, "pass"=w118, "TestCase in"=w111) -> ("error out"=w114:errorcluster, "TestCase out"=w120:refnum<class "testcase-CSMBroadcast.lvclass">)  [unwired: 6 in]
          }
          n138 = flat-sequence {
            tunnel: w84 -> [w97]
            tunnel: [w96] -> w80
            tunnel: w78 -> [w95]
            tunnel: [w95] -> w77
            tunnel: w75 -> [w94]
            tunnel: w80 -> [w102]
            tunnel: [w101] -> w79
            tunnel: w77 -> [w99]
            tunnel: [w99] -> w76
            frame #0 {
              n139 = call "CSM - Send Message and Wait for Reply.vi"("Target Module"=w94, "State"="Macro: Exit") -> ("error out"=w93:errorcluster)  [unwired: 7 in, 2 out]
              n140 = call <vilib>:"Clear Errors.vi"("error in (no error)"=w93) -> ("error out"=w92:errorcluster)  [unwired: 5 in, 1 out]
              n141 = Merge Errors(w97, w92) -> (w96:errorcluster)
            }
            frame #1 {
              n142 = call "CSM - Drop Broadcast Registry.vi"() -> ("error out"=w100:errorcluster)  [unwired: 15 in]
              n143 = Merge Errors(w102, w100) -> (w101:errorcluster)
            }
          }
        }
      }
    }
    frame Disabled {
      # "skip test result while test is under development"
      n144 = call <vilib>:"skip.vi"("error in (no error)"=w415, "TestCase in"=w418) -> ("error out"=w417:errorcluster, "TestCase out"=w416:refnum<class "testcase-CSMBroadcast.lvclass">)  [unwired: 8 in]
    }
  }
  "error out" <- w3
  "TestCase out" <- w1
